vi "CTRE_Phoenix_MotorControl_BufferedTrajectoryPointStream_Write.vi"   [LabVIEW 2018]
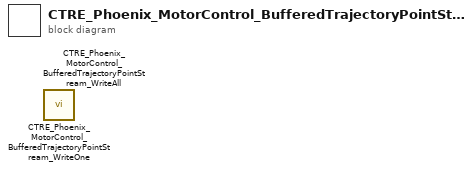
[diagram p0: block diagram]
diagram:
  n1 = call <vilib>:"CTRE_Phoenix_MotorControl_BufferedTrajectoryPointStream_WriteOne.vi"() -> ()  [unwired: 10 in, 2 out]
  n2 = call <vilib>:"CTRE_Phoenix_MotorControl_BufferedTrajectoryPointStream_WriteAll.vi"() -> ()  [unwired: 10 in, 2 out]
